vi "Scale 8 Bit.vi"(8 "error in (no error)":errorcluster, 11 "Data Scaling in":refnum<class "Data Scaling.lvclass">) -> (0 "error out":errorcluster, 3 "Data Scaling out":refnum<class "Data Scaling.lvclass">)   [LabVIEW 2020, in "Unit Tests.lvlib" / "Data Scaling.lvclass"]
uses:
  Data Scaling.lvclass
  Frames & Messages/TypeDefs/Scaling Information.ctl
  <vilib>/addons/_JKI Toolkits/Caraya/classes/Test/Test.lvclass
  <vilib>/addons/_JKI Toolkits/Caraya/classes/Assert/Assert.lvclass
  BCI-1553 API.lvlib
panel:
  out "x .or. y?":u64 format="%064b"
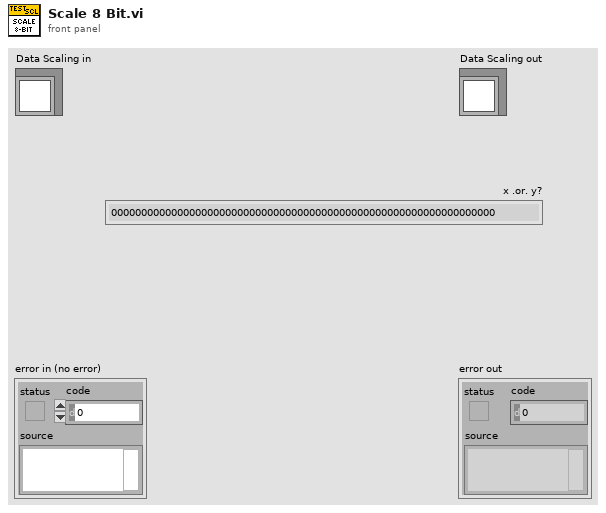
[diagram p1: front panel]
types:
  T1 = typedef "BCI-1553 API.lvlib/Scaling Information.ctl" = cluster{"Bit Offset":i32, "Bit Count":i32, "LSB Resolution":dbl, "2's Complement":bool, "Big Endian":bool, "Sign Bit":bool}
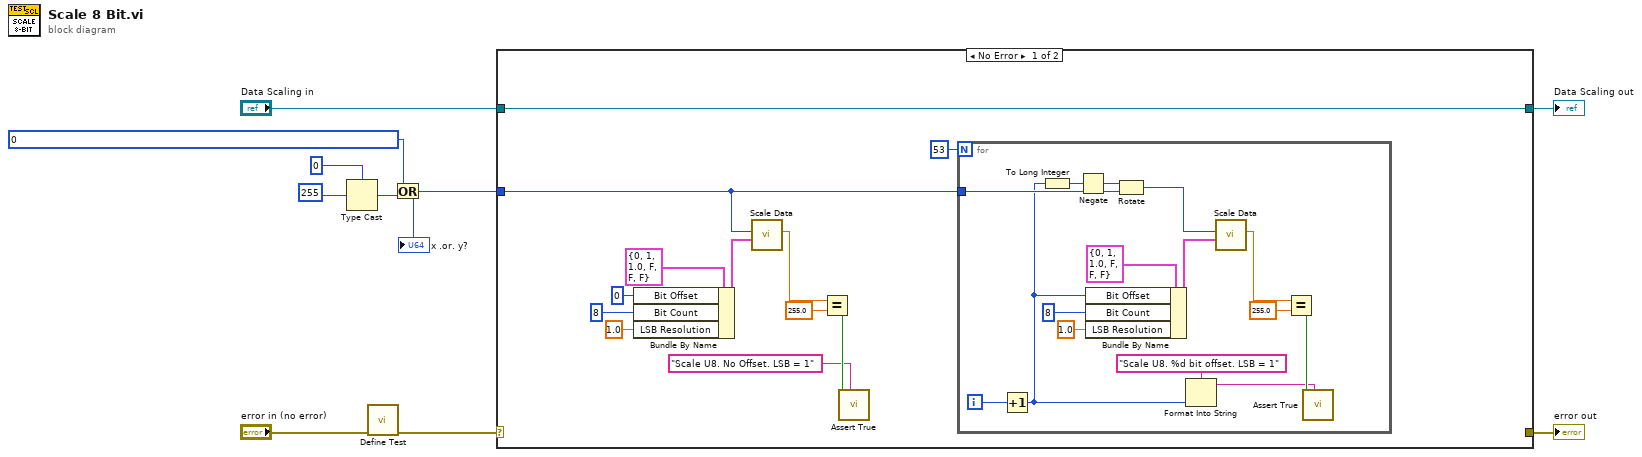
[diagram p0: block diagram]
diagram:
  n1 = Type Cast(type=u64 0 ("unsigned 64bit integer"), x=u8 255 ("unsigned 8bit integer")) -> (*(type *) &x=w2:u64)
  n2 = call <vilib>:"Define Test.vi"("error in (no error)"="error in (no error)") -> ("error out"=w6:errorcluster)  [unwired: 9 in, 1 out]
  n3 = Or(x=u64 0 ("Raw Value"), y=w2) -> (x .or. y?=w5:u64)
  "x .or. y?" <- w5
  n4 = case shown="No Error" w6 {
    selector: w6 -> [_ w39]
    tunnel: [_ w39] -> w10
    tunnel: [w22 w38] -> w8
    tunnel: "Data Scaling in" -> [w22 w38]
    tunnel: w5 -> [w21 _]
    frame No Error {
      n5 = Bundle By Name(cluster=T1 {"Bit Offset"=0, "Bit Count"=1, "LSB Resolution"=1.0, "2's Complement"=FALSE, "Big Endian"=FALSE, "Sign Bit"=FALSE} ("Scaling Info"), "Bit Offset"=0, "Bit Count"=8, "LSB Resolution"=1.0) -> (w16:T1)
      n6 = call "Scale Data.vi"("Scaling Info"=w16, "Raw Value"=w21) -> ("Scaled Value"=w15:dbl)  [unwired: 8 in, 1 out]
      n7 = Equal?(x=w15, y=255.0) -> (x = y?=w13:bool)
      n8 = call <vilib>:"Assert True.vi"("Label"="Scale U8. No Offset. LSB = 1", "True?"=w13) -> ()  [unwired: 8 in, 2 out]
      n9 = for {
        N: 53 -> [_]
        tunnel: w21 -> [w30]
        i -> [w28]
        n10 = Increment(x=w28) -> (x+1=w25:i32)
        n11 = To Long Integer(number=w25) -> (32bit integer=w23:i32)
        n12 = Negate(x=w23) -> (-x=w24:i32)
        n13 = Bundle By Name(cluster=T1 {"Bit Offset"=0, "Bit Count"=1, "LSB Resolution"=1.0, "2's Complement"=FALSE, "Big Endian"=FALSE, "Sign Bit"=FALSE} ("Scaling Info"), "Bit Offset"=w25, "Bit Count"=8, "LSB Resolution"=1.0) -> (w34:T1)
        n14 = Rotate(1:w30, 2:w24) -> (0:w29:u64)
        n15 = Format Into String(format string="Scale U8. %d bit offset. LSB = 1" ("Label"), w25) -> (resulting string=w26:string)  [unwired: 2 in, 1 out]
        n16 = call "Scale Data.vi"("Scaling Info"=w34, "Raw Value"=w29) -> ("Scaled Value"=w35:dbl)  [unwired: 8 in, 1 out]
        n17 = Equal?(x=w35, y=255.0) -> (x = y?=w37:bool)
        n18 = call <vilib>:"Assert True.vi"("Label"=w26, "True?"=w37) -> ()  [unwired: 8 in, 2 out]
      }
    }
    frame Error {
    }
  }
  "error out" <- w10
  "Data Scaling out" <- w8
